vi "comms_Serial_Read_Fixed_Packet.vi"(8 "error in":errorcluster, 10 "Packet Size (Bytes)":u32=1024, 11 "VISA resource in":refnum<visa-resource-name>) -> (0 "error out":errorcluster, 1 "Bytes_In_Buffer":u32, 2 "Data Out":string, 3 "VISA resource Out":refnum<visa-resource-name>, 4 "Bytes Read":u32)   [LabVIEW 2018]
panel:
  out "bytes read":u32
  # "s"
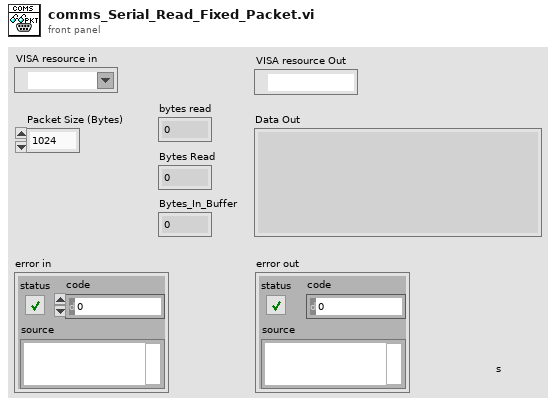
[diagram p1: front panel]
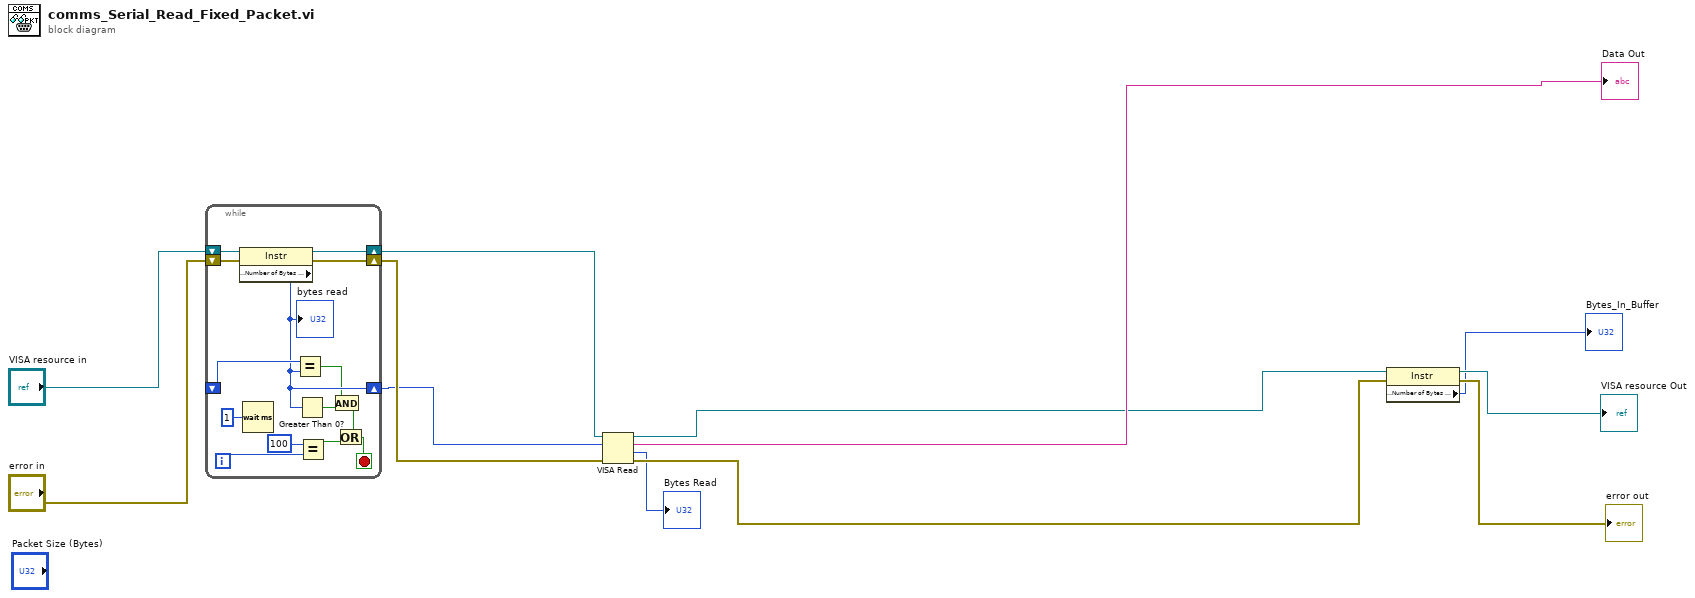
[diagram p0: block diagram]
diagram:
  n1 = while {
    shift-right: [w23] -> w3
    shift-left: "VISA resource in" -> [w26]
    shift-right: [w24] -> w4
    shift-left: "error in" -> [w25]
    shift-right: [w20] -> w1
    shift-left: _ -> [w21]
    i -> [w17]
    stop <- w15 stop-if-true
    n2 = property class="Instr"(reference=w26, error in=w25) -> (reference out=w23:refnum<visa-resource-name>, error out=w24:errorcluster, "Serial Settings:Number of Bytes at Serial Port"=w20:u32)
    "bytes read" <- w20
    n3 = Wait (ms)(milliseconds to wait=u32 1) -> ()  [unwired: 1 out]
    n4 = Equal?(x=w21, y=w20) -> (x = y?=w18:bool)
    n5 = Greater Than 0?(x=w20) -> (x > 0?=w19:bool)
    n6 = Equal?(x=u32 100 ("milliseconds to wait"), y=w17) -> (x = y?=w13:bool)
    n7 = And(x=w18, y=w19) -> (x .and. y?=w14:bool)
    n8 = Or(x=w14, y=w13) -> (x .or. y?=w15:bool)
  }
  n9 = VISA Read(VISA resource name=w3, byte count=w1, error in (no error)=w4) -> (VISA resource name out=w7:refnum<visa-resource-name>, read buffer=→"Data Out":string, return count=→"Bytes Read":u32, error out=w8:errorcluster)
  n10 = property class="Instr"(reference=w7, error in=w8) -> (reference out=→"VISA resource Out":refnum<visa-resource-name>, error out=→"error out":errorcluster, "Serial Settings:Number of Bytes at Serial Port"=→"Bytes_In_Buffer":u32)
